vi "Page_Service_Config_ReadAll.vi"(6 "ctl references":T1, 8 "error in (no error)":errorcluster, 11 "AB_WebService in":refnum<class "AB_WebService.lvclass">) -> (0 "error out":errorcluster, 3 "AB_WebService out":refnum<class "AB_WebService.lvclass">)   [LabVIEW 2020, in "AB_WebService.lvclass"]
uses:
  <vilib>/AppBuilder/AB_Classes/WebService/AB_WebService.lvclass
  <resource>/Framework/Providers/Builds/AppBuilder/AB_UI_Page_Service_Config_References.ctl
  <vilib>/AppBuilder/AB_Classes/WebService/AB_WebService.lvclass/AB_WebService.ctl
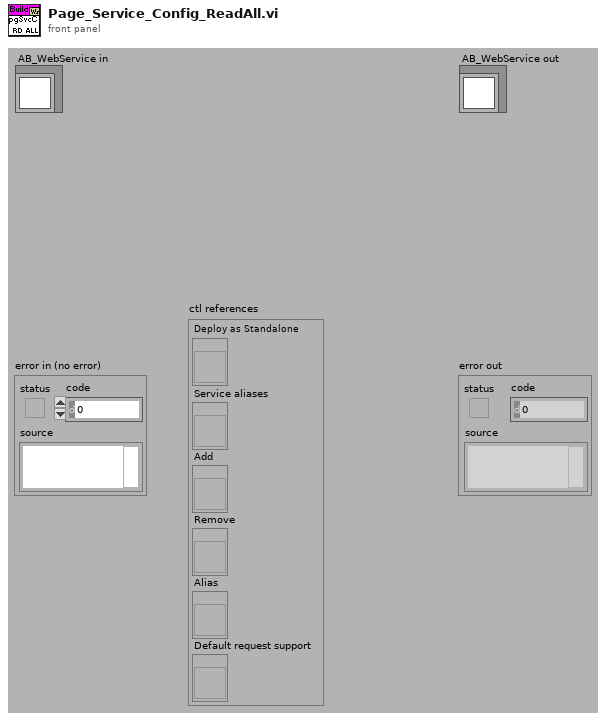
[diagram p1: front panel]
types:
  T1 = typedef "AB_UI_Page_Service_Config_References.ctl" = cluster{"Service aliases":refnum<vi>, "Add":refnum<vi>, "Remove":refnum<vi>, "Alias":refnum<vi>, "Default request support":refnum<vi>, "Deploy as Standalone":refnum<vi>}
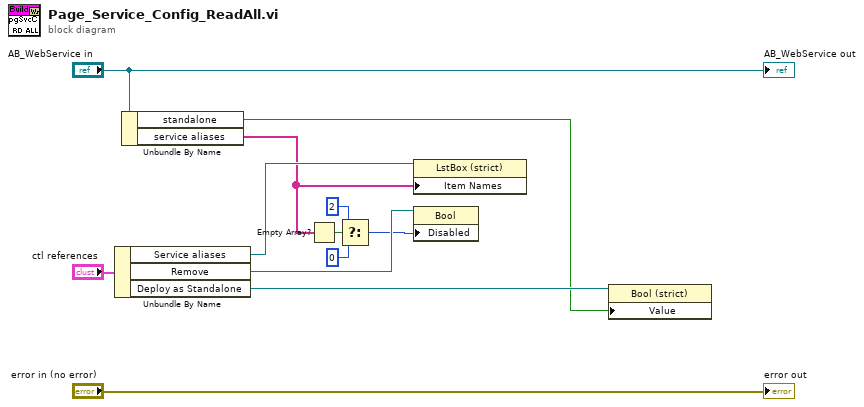
[diagram p0: block diagram]
diagram:
  n1 = Unbundle By Name("ctl references") -> ("Service aliases"=w10:refnum<vi>, "Remove"=w9:refnum<vi>, "Deploy as Standalone"=w2:refnum<vi>)
  n2 = Unbundle By Name("AB_WebService in") -> ("standalone"=w1:bool, "service aliases"=w6:string[])
  n3 = Empty Array?(array=w6) -> (empty?=w5:bool)
  n4 = Select(t=u8 2, s=w5, f=u8 0 ("Disabled")) -> (s? t:f=w4:u8)
  n5 = property class="LstBox (strict)"(reference=w10, "Item Names"=w6) -> ()  [unwired: 1 in, 2 out]
  n6 = property class="Bool"(reference=w9, "Disabled"=w4) -> ()  [unwired: 1 in, 2 out]
  n7 = property class="Bool (strict)"(reference=w2, "Value"=w1) -> ()  [unwired: 1 in, 2 out]
  "error out" <- "error in (no error)"
  "AB_WebService out" <- "AB_WebService in"
